vi "Scan From String.vi"() -> ()   [LabVIEW 2015]
panel:
  in  "input string":string
  out "Has a Driving Licence":bool
  out "Favourite Colour":u32(colorbox)
  out "Date of Birth":timestamp
  out "Name":string
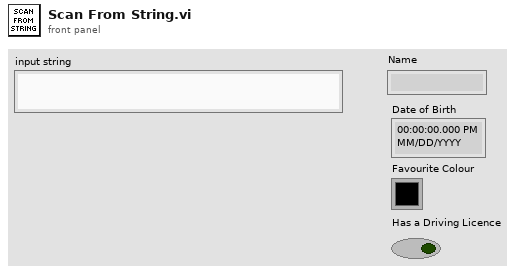
[diagram p1: front panel]
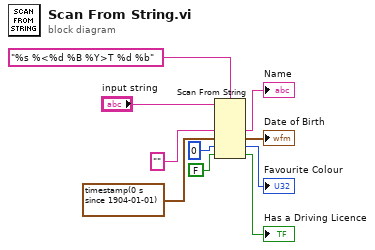
[diagram p0: block diagram]
diagram:
  n1 = Scan From String(format string="%s %<%d %B %Y>T %d %b", input string="input string", default 1="" ("default value 1"), default 2=timestamp(0 s since 1904-01-01) ("default value 2"), default 3=u32 0 ("default value 3"), default 4=FALSE) -> (output 1=→"Name":string, output 2=→"Date of Birth":timestamp, output 3=→"Favourite Colour":u32, output 4=→"Has a Driving Licence":bool)  [unwired: 2 in, 3 out]
